vi "Get Scroll Max.vi"(8 "error in (no error)":errorcluster, 11 "ArrayManager in":refnum<class "ArrayManager.lvclass">) -> (0 "error out":errorcluster, 2 "Scroll Max":i32, 3 "ArrayManager out":refnum<class "ArrayManager.lvclass">)   [LabVIEW 2018, in "OOPanel.lvlib" / "ArrayManager.lvclass"]
uses:
  ArrayManager.lvclass
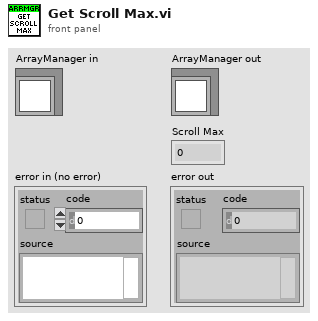
[diagram p1: front panel]
types:
  T1 = typedef "OOPanel.lvlib/ArrayManager.lvclass/UI Refs.ctl" = cluster{"SubPanels":refnum<vi>[], "Scrollbar":refnum<vi>, "Panel VI":refnum<vi>, "Container":refnum<vi>}
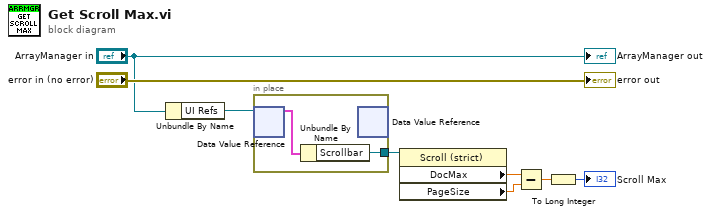
[diagram p0: block diagram]
diagram:
  n1 = Unbundle By Name("ArrayManager in") -> ("UI Refs"=w4:refnum<data-value>)
  n2 = in-place {
    in-place-border: [w9] -> w7
    n3 = in-place-dvr #1(w4) -> (w10:T1)  [unwired: 1 out]
    n4 = Unbundle By Name(w10) -> ("Scrollbar"=w9:refnum<vi>)
    n5 = in-place-dvr #1() -> ()  [unwired: 1 in, 2 out]
  }
  n6 = property class="Scroll (strict)"(reference=w7) -> ("DocMax"=w6:dbl, "PageSize"=w5:dbl)  [unwired: 1 in, 2 out]
  n7 = Subtract(x=w6, y=w5) -> (x-y=w2:dbl)
  n8 = To Long Integer(number=w2) -> (32bit integer=→"Scroll Max":i32)
  "error out" <- "error in (no error)"
  "ArrayManager out" <- "ArrayManager in"
